vi "MonoSpec50 Find Ref Position.vi"(2 "error in":errorcluster, 4 "Moving Ref":refnum<vi>) -> (0 "error out":errorcluster, 1 "Moving":bool caption="Déplacement\nen cours")   [LabVIEW 2019]
doc: "Ce VI envoie un train d'impulsion au moteur, pour le faire tourné dans la direction négative. Les impulsion sont générée en continu jusqu'à ce qu'un front montant soit détecté sur la ligne de détection de position de référence."
uses:
  <vilib>/Utility/error.llb/DialogType.ctl
  <vilib>/DAQmx/write.llb/DAQmx Write (Digital Bool 1Line 1Point).vi
  <vilib>/DAQmx/read.llb/DAQmx Read (Counter U32 1Chan 1Samp).vi
  <vilib>/DAQmx/miscellaneous.llb/DAQmx Fill In Error Info.vi
  <resource>/objmgr/daqmx.rc
panel:
  out "End":bool=TRUE
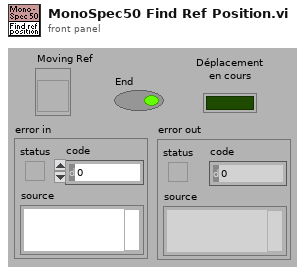
[diagram p1: front panel]
types:
  T1 = typedef "DialogType.ctl" = u16
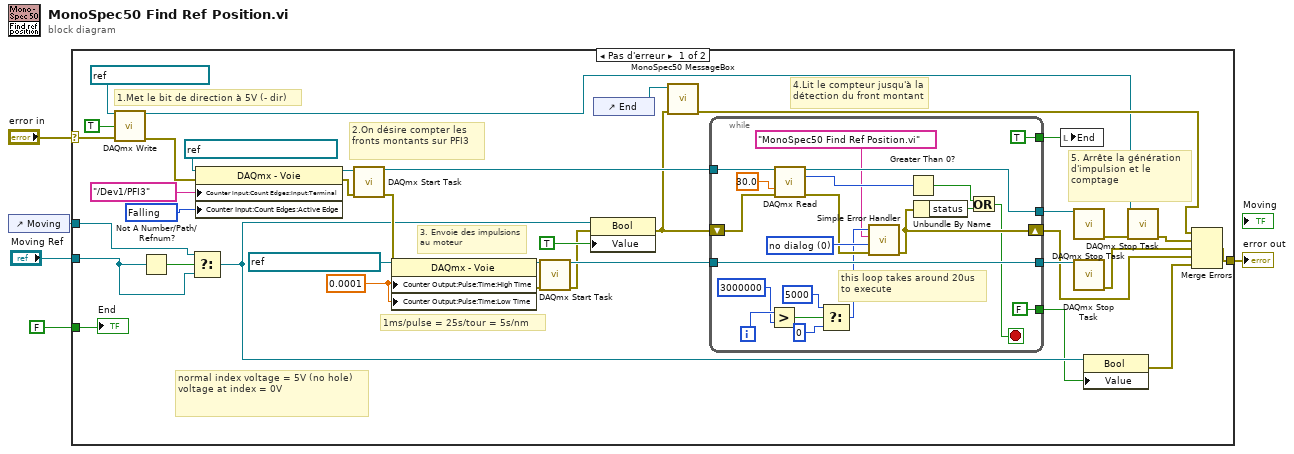
[diagram p0: block diagram]
diagram:
  n1 = control-ref of="Moving"() -> (w2:refnum<vi>)
  n2 = case shown="Pas d'erreur" "error in" {
    selector: "error in" -> [w32 w64]
    tunnel: [w35 w64] -> w4
    tunnel: "Moving Ref" -> [w24 _]
    tunnel: w2 -> [w25 _]
    tunnel: FALSE ("End") -> [w20 _]
    frame No Error {
      w18 = 0.0001 ("CO.Pulse.HighTime")
      w33 = 10171 items=["Rising"=10280, "Falling"=10171] ("CI.CountEdges.ActiveEdge")
      # "normal index voltage = 5V (no hole)\nvoltage at index = 0V"
      # "1ms/pulse = 25s/tour = 5s/nm"
      # "5. Arrête la génération d'impulsion et le comptage"
      # "4.Lit le compteur jusqu'à la détection du front montant"
      # "3. Envoie des impulsions au moteur"
      # "2.On désire compter les fronts montants sur PFI3"
      # "1.Met le bit de direction à 5V (- dir)"
      n3 = call-poly <vilib>:"DAQmx Write.vi"("task/channels in"=refnum<k21> "Direction Spectro", "data"=TRUE, "error in"=w32) -> ("task out"=w13:refnum<k21>, "error out"=w29:errorcluster)  [unwired: 10 in, 1 out]
      n4 = Not A Number/Path/Refnum?(number/path/refnum=w24) -> (NaN/Path/Refnum?=w26:bool)
      n5 = Select(t=w25, s=w26, f=w24) -> (s? t:f=w22:refnum<vi>)
      n6 = property class="DAQmx - Voie"(reference=refnum<k21> "ComptRefPulse Spectro" ("task"), error in=w29, "Counter Input:Count Edges:Input:Terminal"=tag "/Dev1/PFI3" ("CI.CountEdges.Term"), "Counter Input:Count Edges:Active Edge"=w33) -> (reference out=w39:refnum<k21>, error out=w38:errorcluster)
      n7 = call <vilib>:"DAQmx Start Task.vi"("task/channels in"=w39, "error in"=w38) -> ("task out"=w28:refnum<k21>, "error out"=w27:errorcluster)  [unwired: 12 in]
      n8 = property class="DAQmx - Voie"(reference=refnum<k21> "Sortie Pulse Spectro" ("task/channels in"), error in=w27, "Counter Output:Pulse:Time:High Time"=w18, "Counter Output:Pulse:Time:Low Time"=w18) -> (reference out=w8:refnum<k21>, error out=w6:errorcluster)
      n9 = call <vilib>:"DAQmx Start Task.vi"("task/channels in"=w8, "error in"=w6) -> ("task out"=w16:refnum<k21>, "error out"=w7:errorcluster)  [unwired: 12 in]
      n10 = property class="Bool"(reference=w22, error in=w7, "Value"=TRUE) -> (error out=w12:errorcluster)  [unwired: 1 out]
      n11 = control-ref of="End"() -> (w21:refnum<vi>)
      n12 = call <userlib>:"MonoSpec50 MessageBox.vi"("error in (no error)"=w12, "End"=w21) -> ("error out"=w17:errorcluster)  [unwired: 5 in]
      n13 = while {
        tunnel: w28 -> [w63]
        tunnel: [w61] -> w41
        tunnel: w16 -> [w57]
        tunnel: [w57] -> w37
        shift-right: [w51] -> w11
        shift-left: w12 -> [w56]
        tunnel: [TRUE] -> w19
        tunnel: [FALSE ("Value")] -> w9
        i -> [w55]
        stop <- w46 stop-if-true
        w53 = T1 0 items=["no dialog", "OK message", "continue or stop message", "OK message + warnings", "continue/stop + warnings"] ("type of dialog (OK msg:1)")
        # "this loop takes around 20us\nto execute"
        n14 = Greater?(x=w55, y=3000000) -> (0:w50:bool)
        n15 = call-poly <vilib>:"DAQmx Read.vi"("task/channels in"=w63, "timeout"=30.0, "error in"=w56) -> ("task out"=w61:refnum<k21>, "data"=w62:u32, "error out"=w52:errorcluster)  [unwired: 10 in]
        n16 = Select(t=5000 ("error code (no error:0)"), s=w50, f=0) -> (s? t:f=w47:i32)
        n17 = call <vilib>:"Simple Error Handler.vi"("error code (no error:0)"=w47, "error source (\" \")"="MonoSpec50 Find Ref Position.vi" ("error source (\" \")"), "type of dialog (OK msg:1)"=w53, "error in (no error)"=w52) -> ("error out"=w51:errorcluster)  [unwired: 1 in, 4 out]
        n18 = Greater Than 0?(x=w62) -> (x > 0?=w58:bool)
        n19 = Unbundle By Name(w51) -> ("status"=w59:bool)
        n20 = Or(x=w58, y=w59) -> (x .or. y?=w46:bool)
      }
      n21 = local write "End"(w19) -> ()
      n22 = call <vilib>:"DAQmx Stop Task.vi"("task/channels in"=w41) -> ("error out"=w15:errorcluster)  [unwired: 13 in, 1 out]
      n23 = call <vilib>:"DAQmx Stop Task.vi"("task/channels in"=w37) -> ("error out"=w36:errorcluster)  [unwired: 13 in, 1 out]
      n24 = property class="Bool"(reference=w22, "Value"=w9) -> (error out=w10:errorcluster)  [unwired: 1 in, 1 out]
      n25 = call <vilib>:"DAQmx Stop Task.vi"("task/channels in"=w13, "error in"=w15) -> ("error out"=w14:errorcluster)  [unwired: 12 in, 1 out]
      n26 = Merge Errors(w17, w14, w36, w11, w10) -> (w35:errorcluster)
      "End" <- w20
    }
    frame Error {
    }
  }
  "error out" <- w4
